vi "19.04.2025 class2.vi"() -> ()   [LabVIEW 2020]
panel:
  out "min index(es)":i32
  out "min value":dbl
  out "max index(es)":i32
  out "max value":dbl
  in  "Array 4":dbl[](array[numeric])
  out "subarray":dbl[](array[numeric])
  in  "Array 3":dbl[](array[numeric])
  out "concatenated string":string
  out "element":i32[](array[numeric])
  out "appended array":dbl[][][](array[numeric])
  in  "Array 2":dbl[][](array[numeric])
  in  "Array":dbl[][](array[numeric])
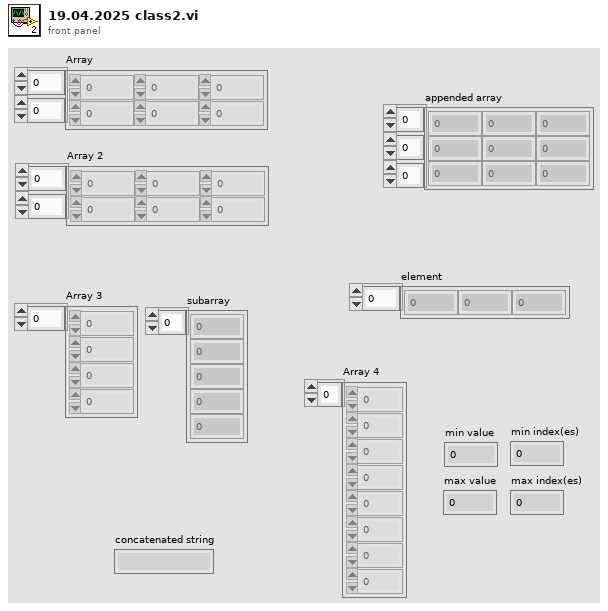
[diagram p1: front panel]
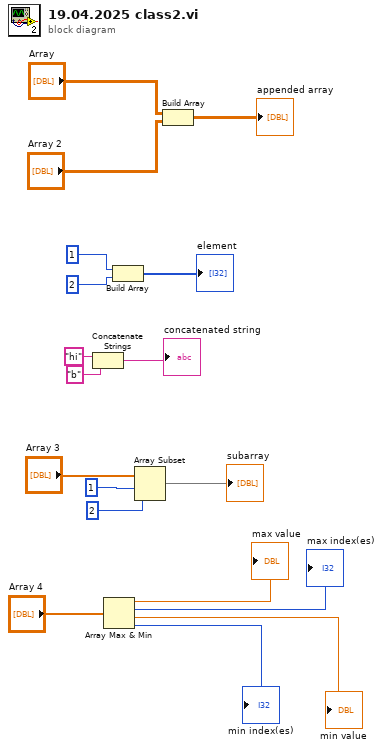
[diagram p0: block diagram]
diagram:
  n1 = Concatenate Strings "Concatenate Strings"("hi" ("string"), "b" ("string")) -> (→"concatenated string":string)
  n2 = Array Max & Min(array="Array 4") -> (max value=→"max value":dbl, max index (indices)=→"max index(es)":i32, min value=→"min value":dbl, min index (indices)=→"min index(es)":i32)
  n3 = Build Array "Build Array"(1, 2) -> (→"element":i32[])
  n4 = Array Subset "Array Subset"(array="Array 3", index=1, length=2) -> (→"subarray":dbl[])
  n5 = Build Array("Array", "Array 2") -> (→"appended array":dbl[][][])
